vi "Aquisicao_NI_paralelo.vi"(4 "rate":dbl=3000.0 format="%0.2f", 5 "error in":errorcluster, 6 "Tempo de Aquisição":dbl, 7 "file path (dialog if empty)":path, 8 "task/channels in":refnum<k21>) -> (0 "error out":errorcluster, 1 "data":dbl[][](array[numeric]) format="%0.2f", 3 "task out":refnum<k21>)   [LabVIEW 2019]
uses:
  <vilib>/DAQmx/read.llb/DAQmx Read (Analog 2D DBL NChan NSamp).vi
  <vilib>/Utility/file.llb/Read Delimited Spreadsheet (string).vi
  <vilib>/Utility/file.llb/Write Delimited Spreadsheet (string).vi
  <vilib>/DAQmx/configure/timing.llb/DAQmx Timing (Sample Clock).vi
  <vilib>/DAQmx/miscellaneous.llb/DAQmx Fill In Error Info.vi
  <vilib>/Utility/file.llb/Write Delimited Spreadsheet (DBL).vi
panel:
  out "Status":string
  out "Slide":u8(slide) scale=0.0..100.0
  out "TimeStamp string":string
  out "Adquirindo":bool
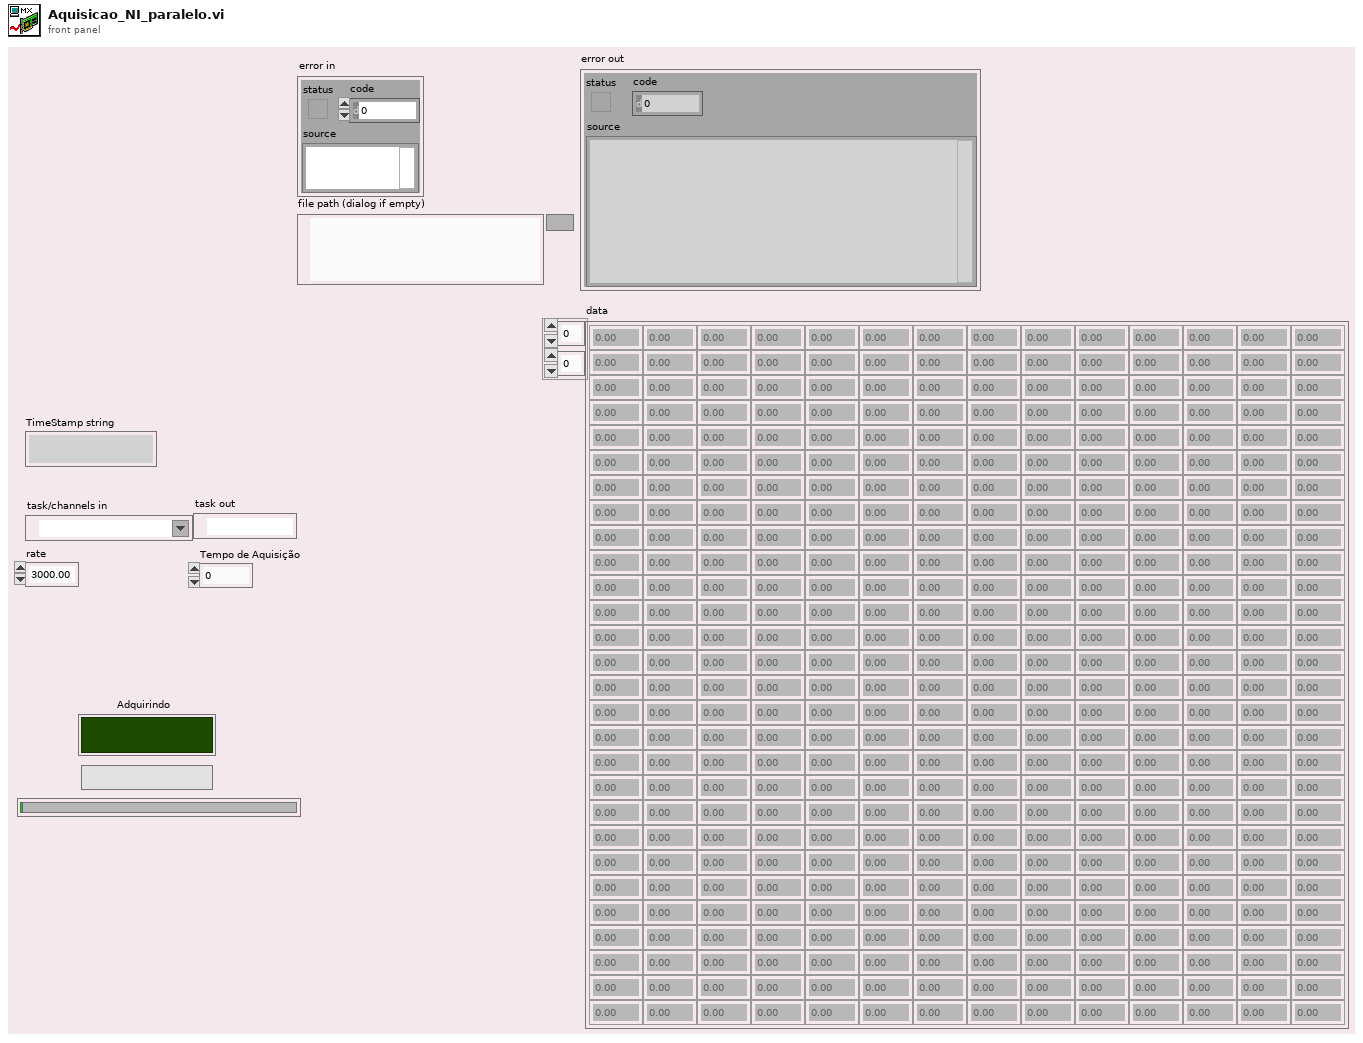
[diagram p1: front panel]
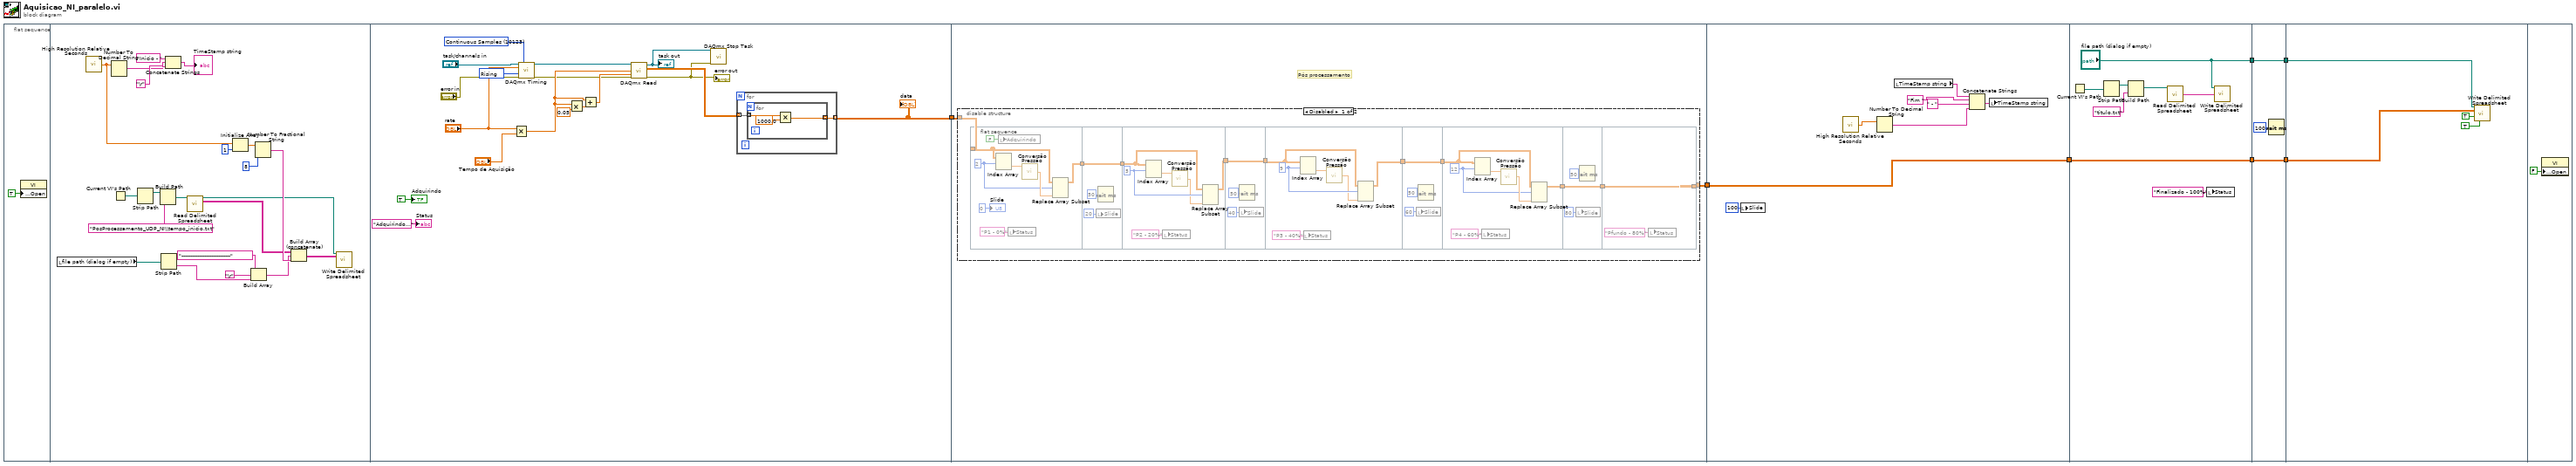
[diagram p0: block diagram]
diagram:
  n1 = flat-sequence {
    tunnel: [w35] -> w2
    tunnel: w2 -> [w54]
    tunnel: [w53] -> w1
    tunnel: [w113] -> w7
    tunnel: w1 -> [w113]
    tunnel: w7 -> [w121]
    tunnel: [w121] -> w6
    tunnel: ["file path (dialog if empty)"] -> w4
    tunnel: w6 -> [w124]
    tunnel: [w124] -> w5
    tunnel: w4 -> [w123]
    tunnel: [w123] -> w3
    tunnel: w5 -> [w125]
    tunnel: w3 -> [w126]
    frame #0 {
      n2 = property class="VI"("Front Panel.Open"=TRUE ("Front Panel Window:Open")) -> ()  [unwired: 2 in, 2 out]
    }
    frame #1 {
      n3 = local read "file path (dialog if empty)"() -> (w13:path)
      n4 = call <vilib>:"High Resolution Relative Seconds.vi"() -> ("relative seconds"=w15:dbl)
      n5 = Number To Decimal String(number=w15) -> (decimal integer string=w16:string)  [unwired: 1 in]
      n6 = Current VI's Path() -> (path=w18:path)
      n7 = Strip Path(path=w18) -> (stripped path=w17:path)  [unwired: 1 out]
      n8 = Build Path(base path=w17, name or relative path="PosProcessamento_UDP_NI\\tempo_inicio.txt") -> (appended path=w21:path)
      n9 = Strip Path(path=w13) -> (name=w12:string)  [unwired: 1 out]
      n10 = Concatenate Strings("Inicio - " ("string"), w16, "\r") -> (→"TimeStamp string":string)
      n11 = call-poly <vilib>:"Read Delimited Spreadsheet.vi"("file path (dialog if empty)"=w21) -> ("new file path (Not A Path if cancelled)"=w22:path, "all rows"=w14:string[][])  [unwired: 9 in, 4 out]
      n12 = Initialize Array(w15, 1 ("dimension size")) -> (w24:dbl[])
      n13 = Build Array("----------------------------" ("element"), "\r", w12) -> (w9:string[])
      n14 = Number To Fractional String(number=w24, precision (6)=i16 8) -> (F-format string=w25:string[])  [unwired: 2 in]
      n15 = Build Array (concatenate)(w14, w9, w25) -> (w20:string[][])
      n16 = call-poly <vilib>:"Write Delimited Spreadsheet.vi"("file path (dialog if empty)"=w22, "2D data"=w20) -> ()  [unwired: 12 in, 2 out]
    }
    frame #2 {
      w34 = 10280 items=["Rising"=10280, "Falling"=10171] ("active edge")
      w41 = 10123 items=["Finite Samples"=10178, "Continuous Samples"=10123, "Hardware Timed Single Point"=12522] ("sample mode")
      n17 = Multiply(x="rate", y="Tempo de Aquisição") -> (x*y=w44:dbl)
      n18 = call-poly <vilib>:"DAQmx Timing.vi"("task/channels in"="task/channels in", "sample mode"=w41, "rate"="rate", "active edge"=w34, "error in"="error in") -> ("task out"=w36:refnum<k21>, "error out"=w37:errorcluster)  [unwired: 9 in]
      n19 = Multiply(x=w44, y=0.05) -> (x*y=w46:dbl)
      n20 = Add(x=w44, y=w46) -> (x+y=w43:dbl)
      n21 = call-poly <vilib>:"DAQmx Read.vi"("task/channels in"=w36, "number of samples per channel"=w44, "timeout"=w43, "error in"=w37) -> ("task out"=w33:refnum<k21>, "data"=w42:dbl[][], "error out"=w32:errorcluster)  [unwired: 9 in]
      "task out" <- w33
      "error out" <- w32
      n22 = call <vilib>:"DAQmx Stop Task.vi"("task/channels in"=w33, "error in"=w32) -> ()  [unwired: 12 in, 2 out]
      n23 = for {
        tunnel: w42 -> [w49] mode=indexing
        tunnel: [w48] -> w35 mode=indexing
        n24 = for {
          tunnel: w49 -> [w52] mode=indexing
          tunnel: [w50] -> w48 mode=indexing
          n25 = Multiply(x=w52, y=1000.0) -> (x*y=w50:dbl)
        }
      }
      "data" <- w35
      "Adquirindo" <- TRUE ("Adquirindo")
      "Status" <- "Adquirindo..." ("Status")
    }
    frame #3 {
      # "Pós processamento"
      n26 = disable-structure shown="Disabled" {
        disable-tunnel: w54 -> [w56 w105]
        disable-tunnel: [w55 w105] -> w53
        frame Disabled {
          n27 = flat-sequence {
            tunnel: w56 -> [w68]
            tunnel: [w69] -> w64
            tunnel: w64 -> [w75]
            tunnel: [w75] -> w63
            tunnel: w63 -> [w78]
            tunnel: [w77] -> w62
            tunnel: w62 -> [w84]
            tunnel: [w84] -> w61
            tunnel: w61 -> [w87]
            tunnel: [w86] -> w60
            tunnel: w60 -> [w93]
            tunnel: [w93] -> w59
            tunnel: w59 -> [w95]
            tunnel: [w97] -> w58
            tunnel: w58 -> [w102]
            tunnel: [w102] -> w57
            tunnel: [w104] -> w55
            tunnel: w57 -> [w104]
            frame #0 {
              w70 = 2 ("disabled index (col)")
              n28 = Index Array(array=w68, index (row)=w70) -> (element=w71:dbl[])  [unwired: 1 in]
              n29 = local write "Adquirindo"(FALSE ("Adquirindo")) -> ()
              n30 = local write "Status"("P1 - 0%" ("Status")) -> ()
              n31 = call "Conversão Pressão.vi"("input"=w71) -> ("output"=w72:dbl[])  [unwired: 2 in]
              n32 = Replace Array Subset(array=w68, new element=w72, index (row)=w70) -> (w69:dbl[][])  [unwired: 1 in]
              "Slide" <- u8 0 ("Slide")
            }
            frame #1 {
              n33 = local write "Slide"(u8 20 ("Slide")) -> ()
              n34 = Wait (ms)(milliseconds to wait=u32 50) -> ()  [unwired: 1 out]
            }
            frame #2 {
              w81 = 5 ("disabled index (col)")
              n35 = Index Array(array=w78, index (row)=w81) -> (element=w80:dbl[])  [unwired: 1 in]
              n36 = local write "Status"("P2 - 20%" ("Status")) -> ()
              n37 = call "Conversão Pressão.vi"("input"=w80) -> ("output"=w79:dbl[])  [unwired: 2 in]
              n38 = Replace Array Subset(array=w78, new element=w79, index (row)=w81) -> (w77:dbl[][])  [unwired: 1 in]
            }
            frame #3 {
              n39 = Wait (ms)(milliseconds to wait=u32 50) -> ()  [unwired: 1 out]
              n40 = local write "Slide"(u8 40 ("Slide")) -> ()
            }
            frame #4 {
              w90 = 9 ("disabled index (col)")
              n41 = Index Array(array=w87, index (row)=w90) -> (element=w89:dbl[])  [unwired: 1 in]
              n42 = local write "Status"("P3 - 40%" ("Status")) -> ()
              n43 = call "Conversão Pressão.vi"("input"=w89) -> ("output"=w88:dbl[])  [unwired: 2 in]
              n44 = Replace Array Subset(array=w87, new element=w88, index (row)=w90) -> (w86:dbl[][])  [unwired: 1 in]
            }
            frame #5 {
              n45 = local write "Slide"(u8 60 ("Slide")) -> ()
              n46 = Wait (ms)(milliseconds to wait=u32 50) -> ()  [unwired: 1 out]
            }
            frame #6 {
              w98 = 12 ("disabled index (col)")
              n47 = Index Array(array=w95, index (row)=w98) -> (element=w96:dbl[])  [unwired: 1 in]
              n48 = local write "Status"("P4 - 60%" ("Status")) -> ()
              n49 = call "Conversão Pressão.vi"("input"=w96) -> ("output"=w99:dbl[])  [unwired: 2 in]
              n50 = Replace Array Subset(array=w95, new element=w99, index (row)=w98) -> (w97:dbl[][])  [unwired: 1 in]
            }
            frame #7 {
              n51 = local write "Slide"(u8 80 ("Slide")) -> ()
              n52 = Wait (ms)(milliseconds to wait=u32 50) -> ()  [unwired: 1 out]
            }
            frame #8 {
              n53 = local write "Status"("Pfundo - 80%" ("Status")) -> ()
            }
          }
        }
        frame Enabled {
        }
      }
    }
    frame #4 {
      n54 = local write "Slide"(u8 100 ("Slide")) -> ()
      n55 = call <vilib>:"High Resolution Relative Seconds.vi"() -> ("relative seconds"=w108:dbl)
      n56 = Number To Decimal String(number=w108) -> (decimal integer string=w107:string)  [unwired: 1 in]
      n57 = local read "TimeStamp string"() -> (w111:string)
      n58 = Concatenate Strings(w111, "Fim " ("string"), " - " ("string"), w107) -> (w112:string)
      n59 = local write "TimeStamp string"(w112) -> ()
    }
    frame #5 {
      n60 = Current VI's Path() -> (path=w119:path)
      n61 = Strip Path(path=w119) -> (stripped path=w120:path)  [unwired: 1 out]
      n62 = Build Path(base path=w120, name or relative path="titulo.txt") -> (appended path=w118:path)
      n63 = call-poly <vilib>:"Read Delimited Spreadsheet.vi"("file path (dialog if empty)"=w118) -> ("first row"=w115:string[])  [unwired: 9 in, 5 out]
      n64 = local write "Status"("Finalizado - 100%" ("Status")) -> ()
      n65 = call-poly <vilib>:"Write Delimited Spreadsheet.vi"("file path (dialog if empty)"="file path (dialog if empty)", "1D data"=w115) -> ()  [unwired: 12 in, 2 out]
    }
    frame #6 {
      n66 = Wait (ms)(milliseconds to wait=u32 100) -> ()  [unwired: 1 out]
    }
    frame #7 {
      n67 = call-poly <vilib>:"Write Delimited Spreadsheet.vi"("file path (dialog if empty)"=w126, "2D data"=w125, "append to file? (new file:F)"=TRUE, "transpose? (no:F)"=TRUE) -> ()  [unwired: 10 in, 2 out]
    }
    frame #8 {
      n68 = property class="VI"("Front Panel.Open"=FALSE ("Front Panel Window:Open")) -> ()  [unwired: 2 in, 2 out]
    }
  }
